vi "AppClose.vi"(8 "error in (no error)":errorcluster) -> ()   [LabVIEW 2016]
uses:
  tools/Translator/Translator.Control.Fglb.Action.vi
  tools/Translator/Translator.Message.ctl
  tools/EventLog/EventLog.Buffer.Action.ctl
  Global/ApplicationGlobal.vi
  tools/Translator/Translator.Global.vi
  tools/EventLog/EventLog.New(single).vi
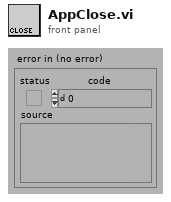
[diagram p1: front panel]
types:
  T1 = typedef "Translator.Control.Fglb.Action.vi" = enum16{"init", "set", "get", "clear"}
  T2 = typedef "Translator.Message.ctl" = enum16{"-", "Event confirmed", "Log out", "Log in", "Shutdown", "Cancel", "Start", "Begin time", "End time", "Duration", "Service Mode", "Ignore Results", "Serial Format", "On", "Off", "OK", "NOK", "NOK %s", "Home", "Work", "Close", "Open", "In progress...", "Missing", "Empty", "Hardware failure", "Initial", "Default", "Total", "Out of range", "Free disk space is below 1GB - contact technician", "Error %d >> %s", "Error %d >> %s >> %s", "Msg %d >> %s", "Laser msg %d %s", "Laser cmd error %s %d", "Laser cmd failed %s", "Laser cmd warning %s", "Laser disconnected", "Laser status %s", "Laser already started", "Laser job unkonwn %s", "Laser job missing %s", "Laser job select failure %s", "Unable to start laser printing (%s)", "Unable to stop laser printing (%s)", "Laser marking aborted", "Laser marking timeout", "Unable to reset Laser Interlock (%s)", "Unable to trigger Laser. Laser not ready (%s)", "Laser job '%s' coordinates not configured", "Starting %s", "Quitting %s", "Configured", "Initializing", "Quitting", "Loading", "Loaded %d results", "Loaded %d events", "Running", "Stopped", "Summary", "Laser", "Do you want to continue?", "Do you want to delete the configuration?", "The configuration is being used by an order. Unable to delete!", "Press confirm button", "Station is not based. Do you want to exit?", "Station requires changeover. Do you want to run the test?", "Test options are not set as default. Do you want to continue?", "Formatting of WabcoNo is disabled. Do you want to continue?", "Product not detected. Do you want to continue?", "Product scan failed. Do you want to continue?", "Calibration", "Log out?", "System", "All", "IDLE", "Translating...%s", "Not found", "Alarm %s", "Run", "Skip", "Abort", "Repeat", "Please wait...", "Database disconnected", "Database disconnected - changeover disabled!", "Login to database successful", "Login to database failed: %d; %s", "Unable to check the product status of reference %d - database disconnected", "Unable to set the product status of reference %d - database disconnected", "Variant file backup %s", "Read variant (%s)", "Result", "Station armed!", "Station requires changeover!", "Select reference number...", "EMERGENCY BUTTON - press Control button", "EMERGENCY DOOR - press Control button", "Resetting Emergency...", "Unable to reset safety circuit - Emergency Button pressed", "Unable to reset safety circuit - Emergency Side Door open", "Station not based", "Station based", "Station not empty", "Station basing...", "No order", "Press Start to begin new order", "Scanning new order", "Order NOK. Correct or scan again", "Order OK. Press Accept", "Order ready", "Revolver incorrect", "Fork incorrect", "Revolver missing", "Revolver empty", "Container missing", "Offline results", "Offline statistics", "Updating statistics %.1f %%", "DMC Configurator", "Door open", "Close the front door", "Press start button", "Done. Open the front door", "Running...", "Running...%.1f %%", "Pause %s", "Pause %s. NOK container missing", "Pause %s. OK container missing", "Pause %s. Revolver empty", "Pause %s. Revolver missing", "Pause %s. Revolver incorrect", "Pause %s. Fork missing", "Pause %s. Fork incorrect", "Pause %s. Too many failures", "Pause %s. Unloading failure", "Pause %s. One slot is not working", "Pause %s. Part order is done. Empty OK container", "Pause %s. Unable to move product to slot", "Pause %s. Unable to move back product pusher", "Pause %s. Unable to lift product", "Pause %s. Unable to move back product lifter", "Pause %s. Unable to move product arm to Work", "Pause %s. Unable to move product arm to NOK", "Pause %s. Unable to move product arm to OK", "Pause %s. Unable to unsuck the NOK product", "Pause %s. Unable to drop the NOK product", "Pause %s. Product OK missing", "Pause %s. Unable to unsuck the OK product", "Pause %s. Unable to drop the OK product", "Stopping...", "File '%s' is missing", "File '%s' is broken", "File '%s' is running", "Log file started (%s)", "Log file ended (%s)", "Log file stopped (%s)", "Log file ignored (%s)", "Log file exported (%s)", "Log file export failed (%s)", "Wrong serial number in log file", "Wrong reference number in log file", "Test steps are missing", "%s = %.3f", "Process param '%s' not found in DB", "Process param '%s' wrong order", "Process param '%s' value %.3f out of limits (%.3f; %.3f)", "Step%d param '%s' not found in DB", "Step%d param '%s' wrong order", "Step%d param '%s' value %.3f out of limits (%.3f; %.3f)", "Step%d EV '%s' not found in DB", "Step%d EV '%s' wrong order", "\"%s\" not found in DB", "\"%s\" wrong order", "\"%s\" value %.3f out of limits (%.3f; %.3f)", "\"%s\" not found in software", "Process init (%s)", "Process started", "Process restarted", "Process run", "Process done", "Process done - remove OK container", "Process aborted", "Process aborted at work", "Process aborted at home", "Process error", "Process error at home", "Process error at work", "Process close", "Process pause", "Process continue", "Process door open", "Process door close", "Process pause at slot %s due to %s", "Select plate from the order to process", "Do you want to start the process?", "Do you want to continue the process?", "There is unfinished order. Do you want to put the new order?", "Product %s %d OK", "Product %s %d NOK", "Unable to unload the slot %s. Product missing in the slot", "Unable to unload the slot %s. Product already in the arm", "Unable to accept the product as OK. Product missing in slot %s", "Unable to accept the product as OK. Product could not drop into the container at slot %s", "Unable to accept the product as NOK. Product could not drop into the container at slot %s", "Scan failed. Error %s", "Scan failed. Scanner disconnected", "Scan failed. Wrong Wabco number %d, limit (%d,%d)", "Scan failed. Wrong serial number %d, limit (%d,%d)", "Scan failed. Wrong date %d, limit (%d,%d)", "Scan failed. Wrong product wabco number %d (expected %d)", "Scan failed. Wrong product serial number %d (expected > 0)", "Scan OK %s", "Scan failed. Unable to determine table position (%s)", "Scan failed. Timeout", "Tune failed. Scanner disconnected", "Tune failed. Timeout", "%s = %d", "%s = %d->%d", "Unable to set %s = %.2f - Air Pressure Inside off", "Unable to set digital output '%s' = %d", "Unable to activate air pressure inside - timeout", "Unable to activate air pressure inside - aborted", "Unable to switch on Air Main Valve - Air Pressure Inlet off", "Unable to switch on Air Main Valve - Door open", "Unable to switch off Air Main Valve - timeout", "Unable to switch off Air Main Valve - aborted", "Unable to rotate Table - timeout", "Unable to rotate Table - aborted", "Unable to rotate Table - Product Move not in Home position", "Unable to rotate Table - Air Pressure Inside off", "Unable to rotate Table - Product Lift A not in Home position", "Unable to rotate Table - Product Lift B not in Home position", "Unable to rotate Table - unlock before movement timeout", "Unable to rotate Table - lock after movement timeout", "Unable to move Table Lock to %s position - timeout", "Unable to move Table Lock to %s position - aborted", "Unable to move Table Lock to %s position - Air Pressure Inside off", "Unable to move Table Lock to %s position - Table not in position", "Unable to move Product Lift A to %s position - timeout", "Unable to move Product Lift B to %s position - timeout", "Unable to move Product Lift A to %s position - aborted", "Unable to move Product Lift B to %s position - aborted", "Unable to move Product Lift A to %s position - Air Pressure Inside off", "Unable to move Product Lift B to %s position - Air Pressure Inside off", "Unable to move Product Lift A to %s position - Table not locked", "Unable to move Product Lift B to %s position - Table not locked", "Unable to move Product Lift A to %s position - Product Arm not in Work position", "Unable to move Product Lift B to %s position - Product Arm not in Work position", "Unable to set Product Suction Gripper %s to %s - timeout", "Unable to set Product Suction Gripper %s to %s - aborted", "Unable to set Product Suction Gripper %s to %s - Air Pressure Inside off", "Unable to set Product Suction Gripper %s to %s - Table slot unkown", "Unable to move Product Arm to %s position - timeout", "Unable to move Product Arm to %s position - aborted", "Unable to move Product Arm to %s position - Air Pressure Inside off", "Unable to move Product Arm to %s position - Product Lift A not in Home position", "Unable to move Product Arm to %s position - Product Lift B not in Home position", "Unable to move Product to %s position - timeout", "Unable to move Product to %s position - aborted", "Unable to move Product to %s position - Air Pressure Inside off", "Unable to move Product to %s position - Table not in position"}
  T3 = enum32{"Invalid", "Standard", "Closed", "Hidden", "Minimized", "Maximized"}
  T4 = typedef "EventLog.Buffer.Action.ctl" = enum16{"init", "re-init", "clear", "set translator", "add", "get", "get unsaved"}
  T5 = typedef "EventLog.EventGui.ctl" = cluster{"ts":dbl, "lev":T6, "usr":i32, "src":T7, "msg":T2, "arg":variant[], "msg_str":string}
  T6 = typedef "EventLog.EventLevel.ctl" = enum8{"Debug", "Info", "Warning", "Error"}
  T7 = typedef "EventLog.EventSource.ctl" = enum16{"All", "Gui", "Ref", "File", "Arch", "Seq", "CPX", "DB", "Laser", "Scan.P", "Scan.O"}
  T8 = cluster{"ts":dbl, "lev":T6, "usr":i32, "src":T7, "msg":T2, "arg":variant[]}
  T9 = typedef "Windows.ExitAction.ctl" = enum16{"Log off from PC", "Shut Down PC", "Reboot PC", "Close Program"}
  T10 = enum32{"invalid app kind", "Development System", "Run Time System", "Student Edition", "Embedded LabVIEW", "Evaluation", "Custom"}
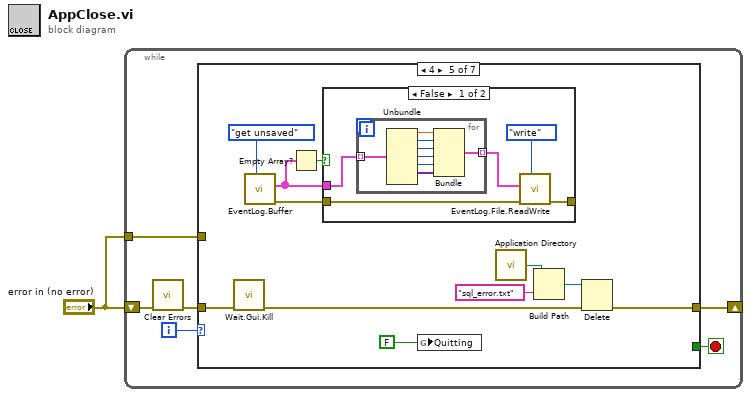
[diagram p0: block diagram]
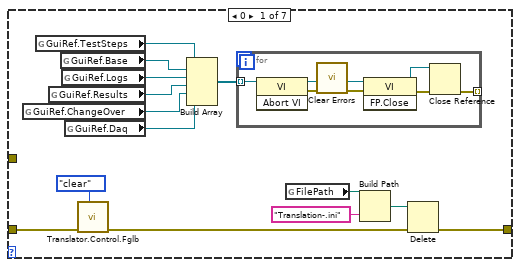
[diagram p2: hidden frame]
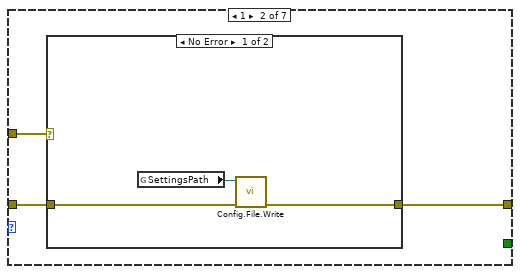
[diagram p3: hidden frame]
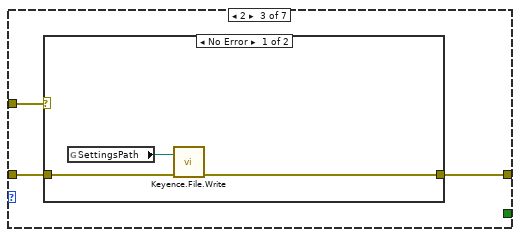
[diagram p5: hidden frame]
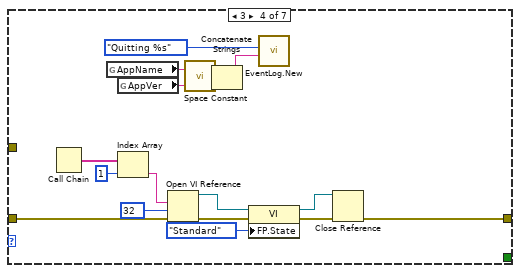
[diagram p7: hidden frame]
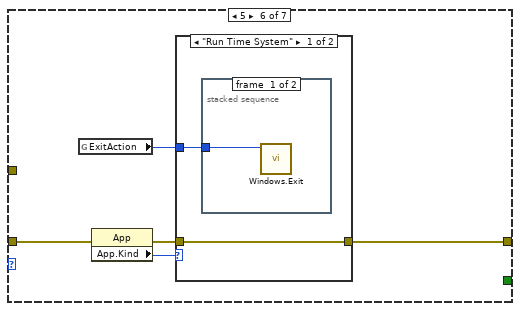
[diagram p9: hidden frame]
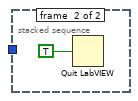
[diagram p10: hidden frame]
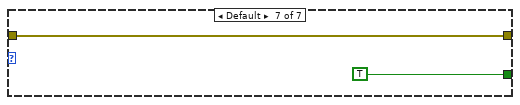
[diagram p12: hidden frame]
diagram:
  n1 = while {
    shift-right: [w3] -> _
    shift-left: "error in (no error)" -> [w5]
    tunnel: "error in (no error)" -> [w2]
    i -> [w7]
    stop <- w6 stop-if-true
    n2 = call <vilib>:"Clear Errors.vi"("error in (no error)"=w5) -> ("error out"=w4:errorcluster)  [unwired: 5 in, 1 out]
    n3 = case shown="4" w7 {
      tunnel: [_ _ _ _ _ _ TRUE] -> w6
      tunnel: w4 -> [w20 w30 w38 w50 w69 w85 w94]
      tunnel: [w8 w31 w37 w49 w60 w84 w94] -> w3
      tunnel: w2 -> [_ w29 w36 _ _ _ _]
      frame 0 {
        n4 = global read "ApplicationGlobal.vi" "GuiRef.ChangeOver"() -> (w15:refnum<vi>)
        n5 = global read "ApplicationGlobal.vi" "GuiRef.TestSteps"() -> (w19:refnum<vi>)
        n6 = global read "ApplicationGlobal.vi" "GuiRef.Results"() -> (w16:refnum<vi>)
        n7 = global read "ApplicationGlobal.vi" "GuiRef.Base"() -> (w18:refnum<vi>)
        n8 = global read "ApplicationGlobal.vi" "GuiRef.Logs"() -> (w17:refnum<vi>)
        n9 = global read "ApplicationGlobal.vi" "GuiRef.Daq"() -> (w14:refnum<vi>)
        n10 = call "Translator.Control.Fglb.vi"("Action"=Translator.Control.Fglb.Action.vi."clear", "error in (no error)"=w20) -> ("error out"=w9:errorcluster)  [unwired: 8 in, 1 out]
        n11 = Build Array(w19, w18, w17, w16, w15, w14) -> (w13:refnum<vi>[])
        n12 = for {
          tunnel: w13 -> [w25] mode=indexing
          tunnel: [w26] -> _ mode=indexing
          n13 = invoke class="VI" method="Abort VI"(reference=w25) -> (reference out=w24:refnum<vi>, error out=w23:errorcluster)  [unwired: 2 in, 1 out]
          n14 = call <vilib>:"Clear Errors.vi"("error in (no error)"=w23) -> ("error out"=w22:errorcluster)  [unwired: 5 in, 1 out]
          n15 = invoke class="VI" method="FP.Close"(reference=w24, error in=w22) -> (reference out=w28:refnum<vi>, error out=w27:errorcluster)  [unwired: 1 in, 1 out]
          n16 = Close Reference(reference=w28, error in (no error)=w27) -> (error out=w26:errorcluster)
        }
        n17 = global read "Translator.Global.vi" "FilePath"() -> (w11:path)
        n18 = Build Path(base path=w11, name or relative path="Translation-.ini") -> (appended path=w10:path)
        n19 = Delete(path (use dialog)=w10, error in=w9) -> (error out=w8:errorcluster)  [unwired: 3 in, 2 out]
      }
      frame 1 {
        n20 = case shown="No Error" w29 {
          tunnel: [w34 w35] -> w31
          tunnel: w30 -> [w33 w35]
          frame No Error {
            n21 = global read "ApplicationGlobal.vi" "SettingsPath"() -> (w32:path)
            n22 = call "Config.File.Write.vi"("error in"=w33, "path"=w32) -> ("error out"=w34:errorcluster)  [unwired: 9 in]
          }
          frame Error {
          }
        }
      }
      frame 2 {
        n23 = case shown="No Error" w36 {
          tunnel: w38 -> [w41 w42]
          tunnel: [w39 w42] -> w37
          frame No Error {
            n24 = global read "ApplicationGlobal.vi" "SettingsPath"() -> (w40:path)
            n25 = call "Keyence.File.Write.vi"("error in"=w41, "segtings path"=w40) -> ("error out"=w39:errorcluster)  [unwired: 9 in]
          }
          frame Error {
          }
        }
      }
      frame 3 {
        n26 = Call Chain() -> (call chain=w53:string[])
        n27 = global read "ApplicationGlobal.vi" "AppName"() -> (w47:string)
        n28 = global read "ApplicationGlobal.vi" "AppVer"() -> (w46:string)
        n29 = Index Array(array=w53, index=1) -> (element=w51:string)
        n30 = Open VI Reference(vi path=w51, options=32, error in (no error)=w50) -> (vi reference=w56:refnum<vi>, error out=w57:errorcluster)  [unwired: 3 in]
        n31 = call <vilib>:"Space Constant.vi"() -> ("String"=w45:string)
        n32 = Concatenate Strings(w47, w45, w46) -> (w44:string)
        n33 = property class="VI"(reference=w56, error in=w57, "FP.State"=T3."Standard" ("Front Panel Window:State")) -> (reference out=w54:refnum<vi>, error out=w55:errorcluster)
        n34 = call-poly "EventLog.New.vi"("Arg"=w44, "Message (-)"=Translator.Message."Quitting %s") -> ()  [unwired: 8 in, 2 out]
        n35 = Close Reference(reference=w54, error in (no error)=w55) -> (error out=w49:errorcluster)
      }
      frame 4 {
        n36 = call "Wait.Gui.Kill.vi"("error in (no error)"=w69) -> ("error out"=w61:errorcluster)  [unwired: 10 in]
        n37 = call "EventLog.Buffer.vi"("action (get)"=EventLog.Buffer.Action."get unsaved") -> ("error out"=w66:errorcluster, "data out"=w65:T5[])  [unwired: 7 in, 2 out]
        n38 = Empty Array?(array=w65) -> (empty?=w64:bool)
        n39 = case shown="False" w64 {
          tunnel: w66 -> [w73 w83]
          tunnel: w65 -> [w71 _]
          tunnel: [w72 w83] -> _
          frame False {
            n40 = for {
              tunnel: w71 -> [w82] mode=indexing
              tunnel: [w75] -> w70 mode=indexing
              n41 = Unbundle(w82) -> ("ts"=w81:dbl, "lev"=w80:T6, "usr"=w78:i32, "src"=w79:T7, "msg"=w77:T2, "arg"=w76:variant[])  [unwired: 1 out]
              n42 = Bundle("ts"=w81, "lev"=w80, "usr"=w78, "src"=w79, "msg"=w77, "arg"=w76) -> (w75:T8)  [unwired: 1 in]
            }
            n43 = call "EventLog.File.ReadWrite.vi"("action (read)"=enum16{"read", "write"}."write", "error in"=w73, "Events in"=w70) -> ("error out"=w72:errorcluster)  [unwired: 4 in, 4 out]
          }
          frame True {
          }
        }
        n44 = global write "ApplicationGlobal.vi" "Quitting"(FALSE ("Quitting")) -> ()
        n45 = call <vilib>:"Application Directory.vi"() -> ("Application Directory"=w59:path)
        n46 = Build Path(base path=w59, name or relative path="sql_error.txt") -> (appended path=w62:path)
        n47 = Delete(path (use dialog)=w62, error in=w61) -> (error out=w60:errorcluster)  [unwired: 3 in, 2 out]
      }
      frame 5 {
        n48 = global read "ApplicationGlobal.vi" "ExitAction"() -> (w86:T9)
        n49 = property class="App"(error in=w85) -> (error out=w87:errorcluster, "App.Kind"=w88:T10)  [unwired: 1 in, 1 out]
        n50 = case shown="\"Run Time System\"" w88 {
          tunnel: w87 -> [w89 w93]
          tunnel: w86 -> [w90 _]
          tunnel: [w89 w93] -> w84
          frame "Run Time System" {
            n51 = stacked-sequence {
              tunnel: w90 -> [w91 _]
              frame #0 {
                n52 = call "Windows.Exit.vi"("Exit Action"=w91) -> ()  [unwired: 6 in, 1 out]
              }
              frame #1 {
                n53 = Quit LabVIEW(quit? (T)=TRUE) -> ()
              }
            }
          }
          frame Default {
          }
        }
      }
      frame Default {
      }
    }
  }
